vi "fpga_Reclaim Control.vi"(7 "reset element? (F)":bool, 10 "reclosing setting":T1={"number of reclosing attempts"=1, "dead times [ms]"=[0, 0, 0, 0, 0, 0, 0], "close pulse duration [ms]"=0, "reclaim time [ms]"=0, "enable synchronism check? (F)"=FALSE, "enable lockout reset? (F)"=FALSE, "lockout reset time [ms]"=0} {"number of reclosing attempts" items=["1"=1, "2"=2, "3"=3, "4"=4, "5"=5, "6"=6, "7"=7]}, 11 "break status? (T)":bool) -> (0 "reclaim time expired?":bool, 3 "reclaim time expired pulse?":bool)   [LabVIEW 2012, in "NI_EP_Protection_FPGA.lvlib"]
uses:
  <vilib>/addons/Electrical Power/Protection/NI_EP_Protection_FPGA.lvlib
  <vilib>/addons/Electrical Power/Protection/Reclosing Logic/subVIs/fpga_Recloser Logic Setting.ctl
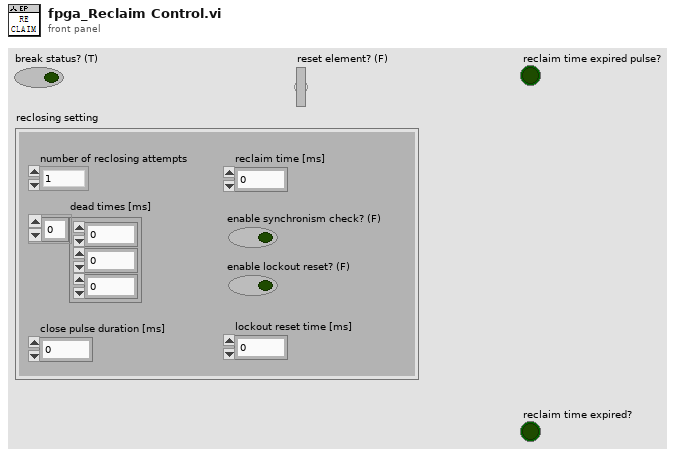
[diagram p1: front panel]
types:
  T1 = typedef "NI_EP_Protection_FPGA.lvlib/fpga_Recloser Logic Setting.ctl" = cluster{"number of reclosing attempts":u8, "dead times [ms]":u32[], "close pulse duration [ms]":u32, "reclaim time [ms]":u32, "enable synchronism check? (F)":bool, "enable lockout reset? (F)":bool, "lockout reset time [ms]":u32}
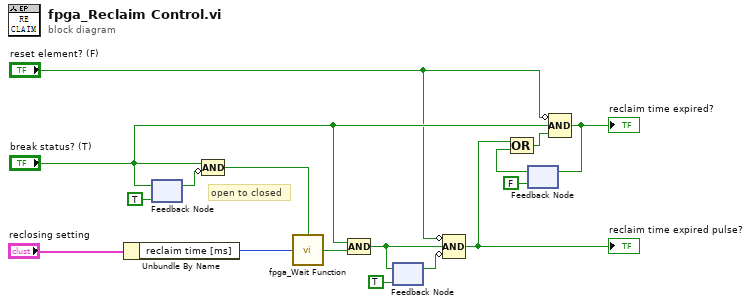
[diagram p0: block diagram]
diagram:
  # "open to closed"
  n1 = Unbundle By Name("reclosing setting") -> ("reclaim time [ms]"=w7:u32)
  n2 = feedback #1(TRUE ("Breaker Status?")) -> (w14:bool)
  n3 = feedback-in #1("break status? (T)") -> ()
  n4 = Compound Arithmetic op=AND("break status? (T)", invert w14) -> (w16:bool)
  n5 = call <vilib>:"fpga_Wait Function.vi"("start? (F)"=w16, "timeout (ms)"=w7) -> ("timeout?"=w15:bool)  [unwired: 13 in]
  n6 = Compound Arithmetic op=AND("break status? (T)", w15) -> (w4:bool)
  n7 = feedback #2(TRUE ("Breaker Status?")) -> (w5:bool)
  n8 = feedback-in #2(w4) -> ()
  n9 = Compound Arithmetic op=AND(invert "reset element? (F)", w4, invert w5) -> (w3:bool)
  "reclaim time expired pulse?" <- w3
  n10 = feedback #3(FALSE) -> (w12:bool)
  n11 = Compound Arithmetic op=OR(w3, w12) -> (w10:bool)
  n12 = Compound Arithmetic op=AND(invert "reset element? (F)", "break status? (T)", w10) -> (w11:bool)
  "reclaim time expired?" <- w11
  n13 = feedback-in #3(w11) -> ()
